vi "Stop IO Tasks.vi"(8 "error in (no error)":errorcluster, 11 "BaseProducer in":refnum<class "BaseProducer.lvclass">) -> (0 "error out":errorcluster, 3 "BaseProducer out":refnum<class "BaseProducer.lvclass">)   [LabVIEW 2013, in "BaseProducer.lvclass"]
doc: "This private method stops the IO tasks for the current experiment. This VI executes normally even if an error occurs before hand."
uses:
  BaseProducer.lvclass
  BaseProducer.lvclass/BaseProducer.ctl
  <vilib>/DAQmx/write.llb/DAQmx Write (Analog 1D DBL NChan 1Samp).vi
  <vilib>/DAQmx/write.llb/DAQmx Write (Digital 1D Bool NChan 1Samp 1Line).vi
  <vilib>/DAQmx/miscellaneous.llb/DAQmx Fill In Error Info.vi
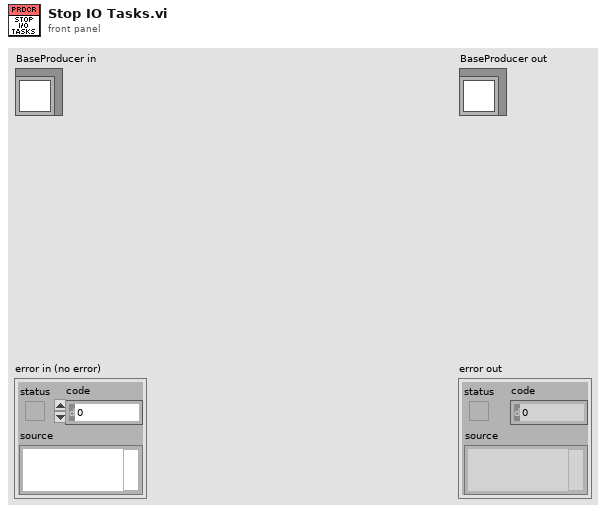
[diagram p1: front panel]
types:
  T1 = typedef "BaseProducer.lvclass/IO Task Cluster.ctl" = cluster{"Dynamic P Tasks":refnum<k21>, "AI Tasks":refnum<k21>, "DIO Tasks":refnum<k21>, "AO Tasks":refnum<k21>}
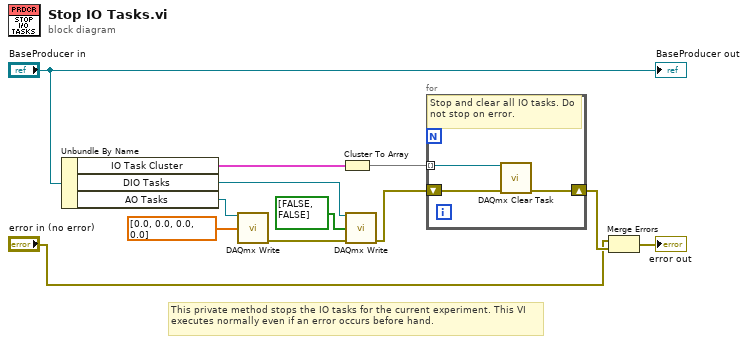
[diagram p0: block diagram]
diagram:
  # "This private method stops the IO tasks for the current experiment. This VI executes normally even if an error occurs before hand."
  n1 = Unbundle By Name("BaseProducer in") -> ("IO Task Cluster"=w11:T1, "DIO Tasks"=w4:refnum<k21>, "AO Tasks"=w6:refnum<k21>)
  n2 = call-poly <vilib>:"DAQmx Write.vi"("task/channels in"=w6, "data"=dbl[] [0.0, 0.0, 0.0, 0.0]) -> ("error out"=w5:errorcluster)  [unwired: 11 in, 2 out]
  n3 = Cluster To Array(cluster=w11) -> (array=w8:refnum<k21>[])
  n4 = call-poly <vilib>:"DAQmx Write.vi"("task/channels in"=w4, "data"=bool[] [FALSE, FALSE], "error in"=w5) -> ("error out"=w2:errorcluster)  [unwired: 10 in, 2 out]
  n5 = for {
    tunnel: w8 -> [w14] mode=indexing
    shift-right: [w15] -> w10
    shift-left: w2 -> [w13]
    # "Stop and clear all IO tasks. Do not stop on error."
    n6 = call <vilib>:"DAQmx Clear Task.vi"("task in"=w14, "error in"=w13) -> ("error out"=w15:errorcluster)  [unwired: 13 in]
  }
  n7 = Merge Errors("error in (no error)", w10) -> (→"error out":errorcluster)
  "BaseProducer out" <- "BaseProducer in"
